vi "Update Robot State.vi"(8 "error in (no error)":errorcluster, 11 "Grips Robot in":refnum<class "Grips Robot.lvclass">) -> (0 "error out":errorcluster, 3 "Grips Robot out":refnum<class "Grips Robot.lvclass">)   [LabVIEW 2013, in "Grips Robot.lvclass"]
uses:
  Grips Robot.lvclass
  Grips Robot.lvclass/Grips Robot.ctl
  Hardware Interface/Hardware Interface.lvclass/Hardware Interface.ctl
  Hardware Interface/Hardware Interface.lvclass
  Helpers/Helpers.lvlib
  <vilib>/ptbypt/NI_PtbyPt.lvlib
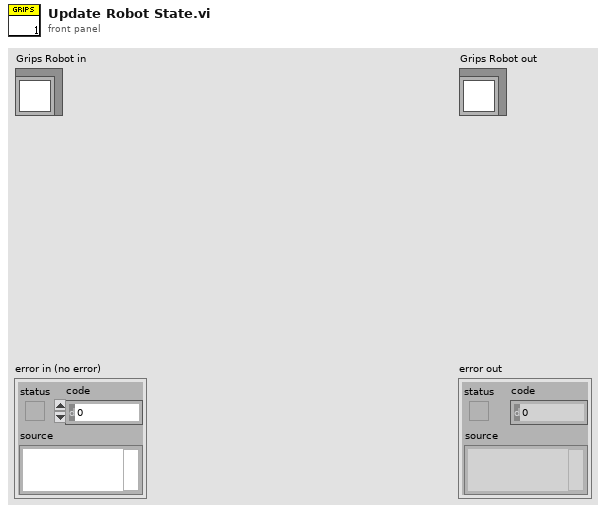
[diagram p1: front panel]
types:
  T1 = typedef "Grips Robot.lvclass/JointState.ctl" = cluster{"header":cluster{"seq":u32, "stamp":cluster{"sec":i32, "nsec":i32}, "frame_id":string}, "name":string[], "position":dbl[], "velocity":dbl[], "effort":dbl[]}
  T2 = typedef "Grips Robot.lvclass/JointMapping.ctl" = cluster{"name":string[], "position":string[], "velocity":string[], "effort":string[], "command":string[]}
  T3 = typedef "Hardware Interface.lvclass/DblArrayWithName.ctl" = cluster{"name":string[], "value":dbl[]}
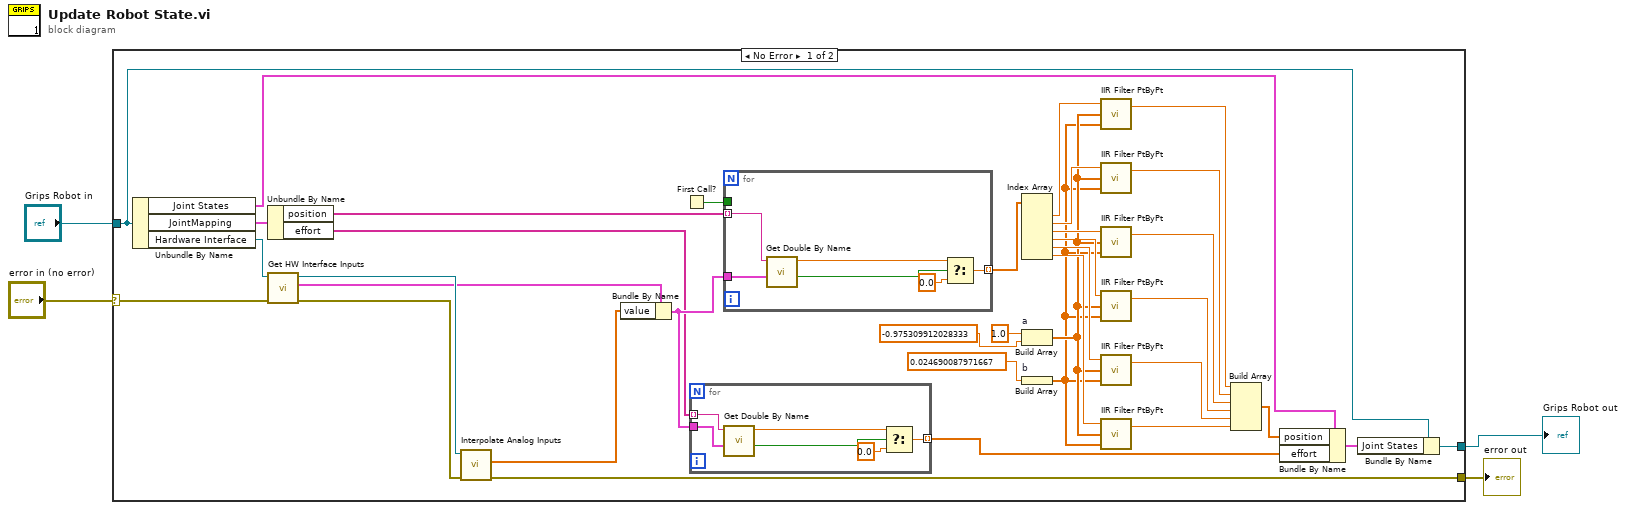
[diagram p0: block diagram]
diagram:
  n1 = case shown="No Error" "error in (no error)" {
    selector: "error in (no error)" -> [w35 w54]
    tunnel: [w32 w54] -> w3
    tunnel: [w39 w53] -> w1
    tunnel: "Grips Robot in" -> [w40 w53]
    frame No Error {
      n2 = Unbundle By Name(w40) -> ("Joint States"=w37:T1, "JointMapping"=w30:T2, "Hardware Interface"=w29:refnum<class "Hardware Interface.lvclass">)
      n3 = Unbundle By Name(w30) -> ("position"=w25:string[], "effort"=w26:string[])
      n4 = call "Get HW Interface Inputs.vi"("error in (no error)"=w35, "Hardware Interface in"=w29) -> ("error out"=w34:errorcluster, "Analog Inputs"=w31:T3, "Hardware Interface out"=w33:refnum<class "Hardware Interface.lvclass">)  [unwired: 6 in, 1 out]
      n5 = call "Interpolate Analog Inputs.vi"("error in (no error)"=w34, "Hardware Interface in"=w33) -> ("error out"=w32:errorcluster, "Interpolated Values"=w36:dbl[])  [unwired: 7 in, 1 out]
      n6 = Bundle By Name(cluster=w31, "value"=w36) -> (w27:T3)
      n7 = First Call?() -> (First Call?: T/F=w24:bool)
      n8 = for {
        tunnel: w27 -> [w45]
        tunnel: w26 -> [w46] mode=indexing
        tunnel: [w42] -> w28 mode=indexing
        n9 = call "Get Double By Name.vi"("name"=w46, "Analog Values"=w45) -> ("result"=w43:dbl, "found?"=w44:bool)  [unwired: 7 in]
        n10 = Select(t=w43, s=w44, f=0.0) -> (s? t:f=w42:dbl)
      }
      n11 = for {
        tunnel: w27 -> [w51]
        tunnel: w25 -> [w52] mode=indexing
        tunnel: w24 -> [_]
        tunnel: [w47] -> w19 mode=indexing
        n12 = call "Get Double By Name.vi"("name"=w52, "Analog Values"=w51) -> ("result"=w50:dbl, "found?"=w49:bool)  [unwired: 7 in]
        n13 = Select(t=w50, s=w49, f=0.0) -> (s? t:f=w47:dbl)
      }
      n14 = Index Array(array=w19) -> (element #1=w20:dbl, element #2=w18:dbl, element #3=w17:dbl, element #4=w16:dbl, element #5=w15:dbl, element #6=w14:dbl)  [unwired: 6 in]
      n15 = Build Array "a"(1.0, -0.975309912028333) -> (w13:dbl[])
      n16 = Build Array "b"(0.024690087971667) -> (w12:dbl[])
      n17 = call <vilib>:"IIR Filter PtByPt.vi"("Forward Coefficients"=w12, "Reverse Coefficients"=w13, "x"=w20) -> ("Filtered x"=w11:dbl)  [unwired: 1 in, 1 out]
      n18 = call <vilib>:"IIR Filter PtByPt.vi"("Forward Coefficients"=w12, "Reverse Coefficients"=w13, "x"=w18) -> ("Filtered x"=w10:dbl)  [unwired: 1 in, 1 out]
      n19 = call <vilib>:"IIR Filter PtByPt.vi"("Forward Coefficients"=w12, "Reverse Coefficients"=w13, "x"=w17) -> ("Filtered x"=w9:dbl)  [unwired: 1 in, 1 out]
      n20 = call <vilib>:"IIR Filter PtByPt.vi"("Forward Coefficients"=w12, "Reverse Coefficients"=w13, "x"=w16) -> ("Filtered x"=w8:dbl)  [unwired: 1 in, 1 out]
      n21 = call <vilib>:"IIR Filter PtByPt.vi"("Forward Coefficients"=w12, "Reverse Coefficients"=w13, "x"=w15) -> ("Filtered x"=w7:dbl)  [unwired: 1 in, 1 out]
      n22 = call <vilib>:"IIR Filter PtByPt.vi"("Forward Coefficients"=w12, "Reverse Coefficients"=w13, "x"=w14) -> ("Filtered x"=w6:dbl)  [unwired: 1 in, 1 out]
      n23 = Build Array(w11, w10, w9, w8, w7, w6) -> (w5:dbl[])
      n24 = Bundle By Name(cluster=w37, "position"=w5, "effort"=w28) -> (w38:T1)
      n25 = Bundle By Name(cluster=w40, "Joint States"=w38) -> (w39:refnum<class "Grips Robot.lvclass">)
    }
    frame Error {
    }
  }
  "error out" <- w3
  "Grips Robot out" <- w1
